vi "LED_Acquire.vi"(8 "error in (no error)":errorcluster, 11 "LED Notifier":refnum<notifier>) -> (0 "error out":errorcluster, 3 "LED Notifier (dup)":refnum<notifier>)   [LabVIEW 2010, in "lib1299.lvlib"]
doc: "This VI starts the acquire LED indication.\n\nInputs:\nLED Notifier - reference to the LED Notifier\nerror in - error input cluster\n\nOutputs:\nLED Notifier (dup) - duplicate of notifier in\nerror out - error output cluster"
uses:
  lib1299.lvlib
  TYP_LEDSegNotifier.ctl
  TYP_LEDCommand.ctl
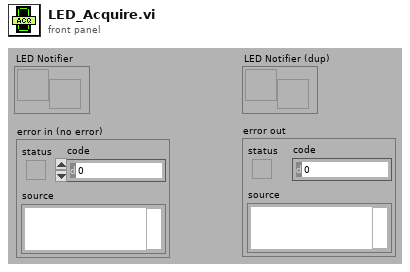
[diagram p1: front panel]
types:
  T1 = typedef "lib1299.lvlib/TYP_LEDSegNotifier.ctl" = cluster{"notification":T2, "Data":i32}
  T2 = typedef "lib1299.lvlib/TYP_LEDCommand.ctl" = enum16{"Init", "Go ACQ", "Go XFR", "Manual", "Stop", "Exit"}
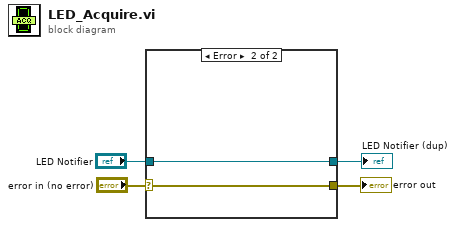
[diagram p0: block diagram]
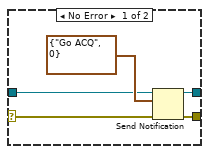
[diagram p2: hidden frame]
diagram:
  n1 = case shown="Error" "error in (no error)" {
    selector: "error in (no error)" -> [w8 w11]
    tunnel: [w9 w11] -> w4
    tunnel: "LED Notifier" -> [w6 w10]
    tunnel: [w5 w10] -> w1
    frame No Error {
      n2 = Send Notification(notification=T1 {"notification"=enum."Go ACQ", "Data"=0} ("LED Display"), notifier=w6, error in (no error)=w8) -> (notifier out=w5:refnum<notifier>, error out=w9:errorcluster)
    }
    frame Error {
    }
  }
  "error out" <- w4
  "LED Notifier (dup)" <- w1
